vi "WebView2LoaderCheck.vi"(5 "Error In":errorcluster) -> (19 "Error Out":errorcluster)   [LabVIEW 2020, in "DP_WebView.lvclass"]
uses:
  DP_WebView.lvclass
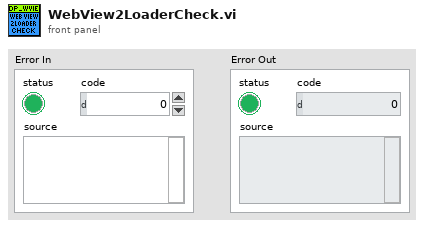
[diagram p1: front panel]
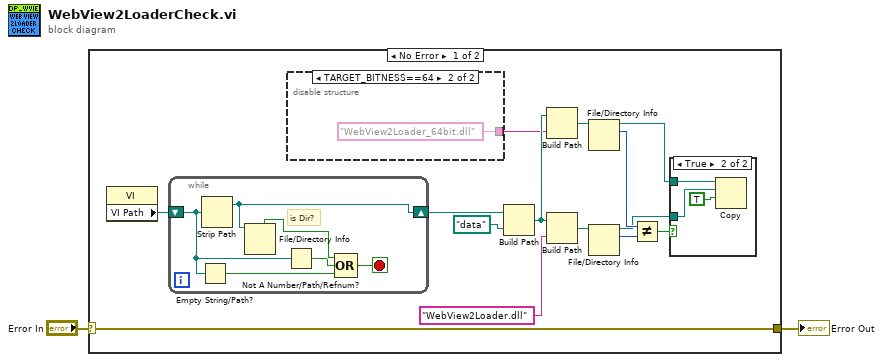
[diagram p0: block diagram]
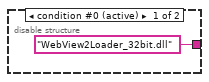
[diagram p3: hidden frame]
diagram:
  n1 = case shown="No Error" "Error In" {
    selector: "Error In" -> [w16 w28]
    tunnel: [w16 w28] -> w1
    frame No Error {
      n2 = property class="VI"() -> ("VI Path"=w15:path)  [unwired: 2 in, 2 out]
      n3 = while {
        shift-right: [w20] -> w14
        shift-left: w15 -> [w22]
        stop <- w24 stop-if-true
        # "is Dir?"
        n4 = Empty String/Path?(string/path=w22) -> (empty?=w21:bool)
        n5 = Strip Path(path=w22) -> (stripped path=w20:path)  [unwired: 1 out]
        n6 = File/Directory Info(path=w20) -> (directory=w25:bool)  [unwired: 1 in, 6 out]
        n7 = Not A Number/Path/Refnum?(number/path/refnum=w22) -> (NaN/Path/Refnum?=w23:bool)
        n8 = Compound Arithmetic op=OR(w25, w23, w21) -> (w24:bool)
      }
      n9 = disable-structure shown="TARGET_BITNESS==64" {
        disable-tunnel: ["WebView2Loader_32bit.dll" "WebView2Loader_64bit.dll"] -> w8
        frame condition #0 (active) {
        }
        frame condition #1 {
        }
      }
      n10 = Build Path(base path=w14, name or relative path=path "data" ("Relative path (.)")) -> (appended path=w9:path)
      n11 = Build Path(base path=w9, name or relative path=w8) -> (appended path=w10:path)
      n12 = Build Path(base path=w9, name or relative path="WebView2Loader.dll") -> (appended path=w11:path)
      n13 = File/Directory Info(path=w10) -> (path out=w4:path, size=w7:i64)  [unwired: 1 in, 5 out]
      n14 = File/Directory Info(path=w11) -> (path out=w3:path, size=w6:i64)  [unwired: 1 in, 5 out]
      n15 = Not Equal?(x=w7, y=w6) -> (x != y?=w5:bool)
      n16 = case shown="True" w5 {
        tunnel: w4 -> [_ w19]
        tunnel: w3 -> [_ w18]
        frame False {
        }
        frame True {
          n17 = Copy(9:TRUE ("overwrite (F)"), 10:w18, 11:w19) -> ()  [unwired: 2 in, 3 out]
        }
      }
    }
    frame Error {
    }
  }
  "Error Out" <- w1
